vi "LeerBD.vi"(8 "error in (no error)":errorcluster) -> (0 "error out":errorcluster, 2 "BD":T1={"niv_presion_son_ref"=97.0, "Incertidumbre"="", "Tol +"="", "Tol -"="", "rangos"=[], "frecuencia_ref"=97.0}, 3 "Prueba07 out":refnum<class "Prueba07.lvclass">)   [LabVIEW 2019, in "Prueba07.lvclass"]
uses:
  Prueba07.lvclass
  BD.ctl
  Base de Datos/SQLiteConnector/SQLiteConnection.lvclass
  Base de Datos/Base de Datos.lvclass
panel:
  out "rangos out":string[][](array[string])
  in  "Tipo Equipo":enum16{"Sonometro", "Calibrador", "Dosimetro"}(ring)
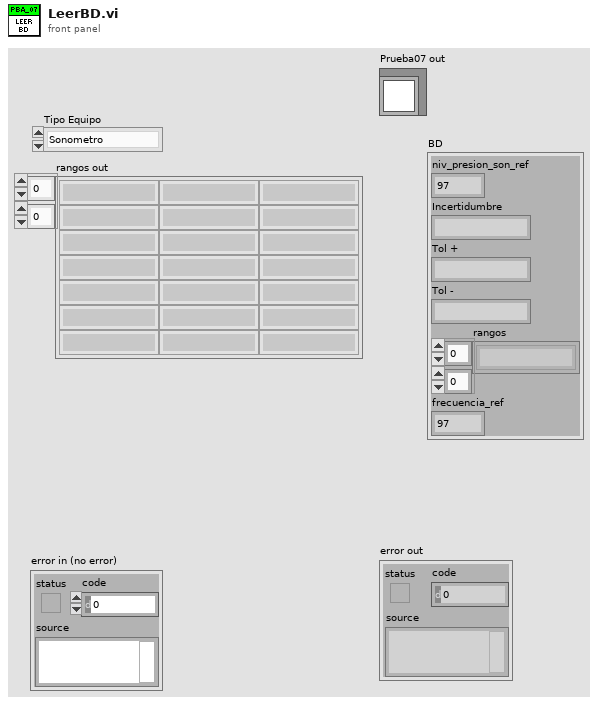
[diagram p1: front panel]
types:
  T1 = typedef "Prueba07.lvclass/BD.ctl" = cluster{"niv_presion_son_ref":dbl, "Incertidumbre":string, "Tol +":string, "Tol -":string, "rangos":string[][], "frecuencia_ref":dbl}
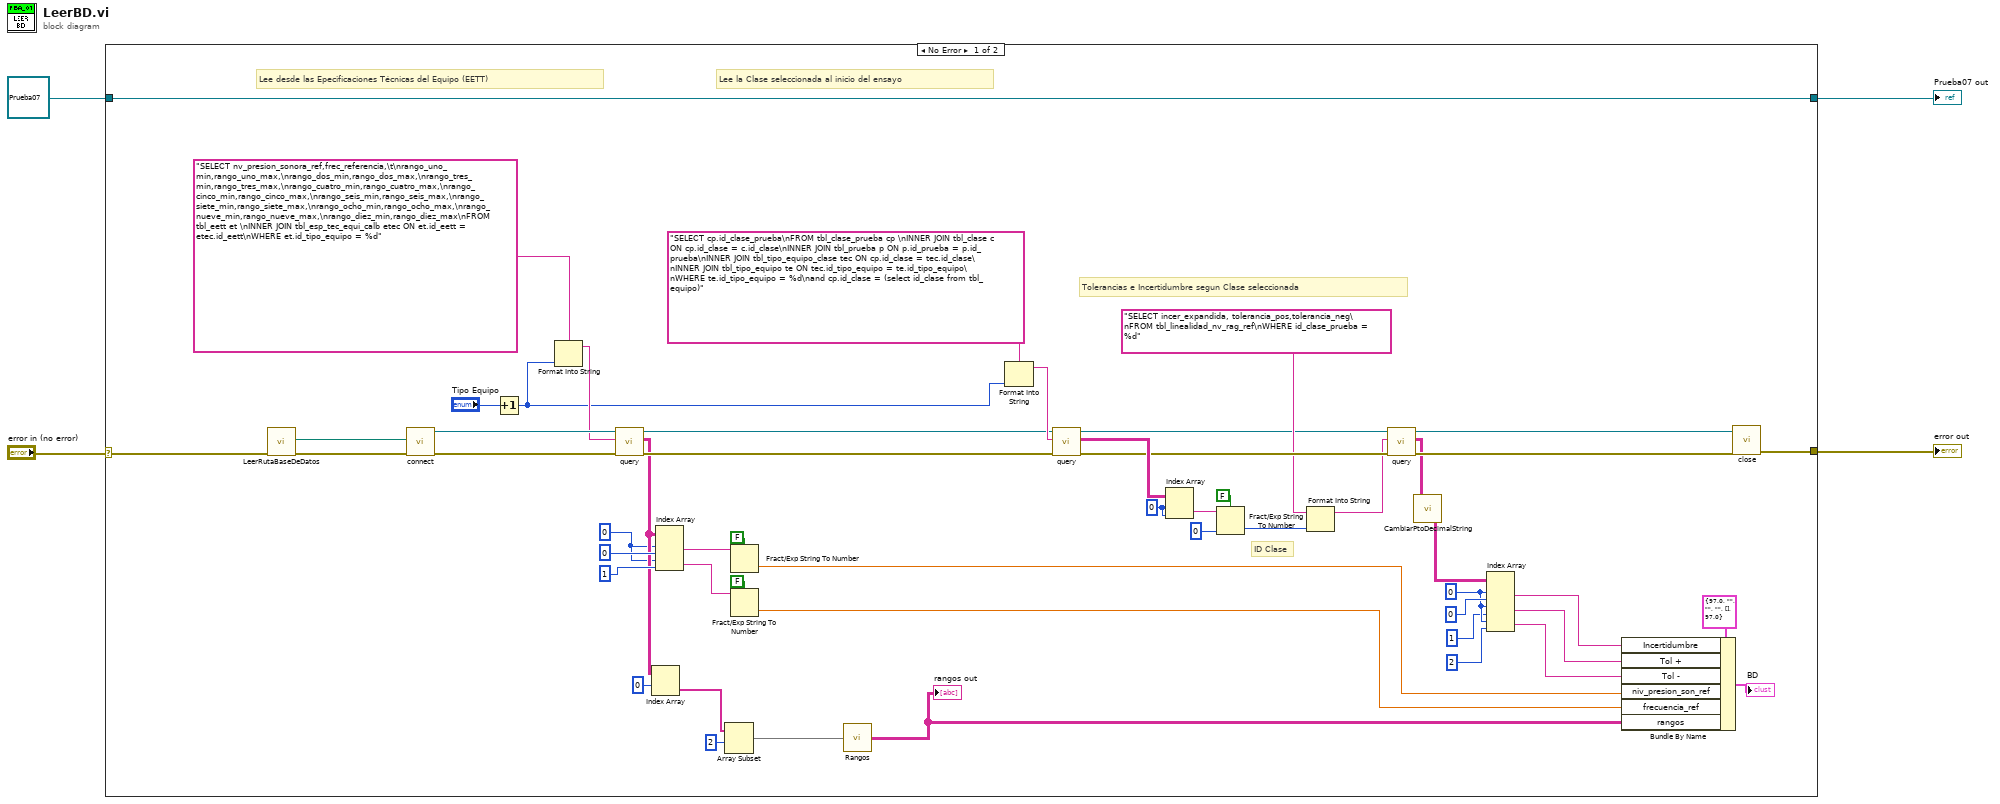
[diagram p0: block diagram]
diagram:
  n1 = case shown="No Error" "error in (no error)" {
    selector: "error in (no error)" -> [w49 w59]
    tunnel: [w35 w59] -> w3
    tunnel: [w57 w58] -> w1
    tunnel: refnum<class "Prueba07.lvclass"> refnum ("Prueba02 in") -> [w57 w58]
    frame No Error {
      w20 = 0 ("index (row)")
      w41 = 0 ("index (row)")
      w7 = 0 ("index (row)")
      # "Tolerancias e Incertidumbre segun Clase seleccionada"
      # "ID Clase"
      # "Lee la Clase seleccionada al inicio del ensayo"
      # "Lee desde las Epecificaciones Técnicas del Equipo (EETT)"
      n2 = call "LeerRutaBaseDeDatos.vi"("error in (no error)"=w49) -> ("error out"=w52:errorcluster, "Database Path"=w51:path)  [unwired: 9 in]
      n3 = call "connect.vi"("error in (no error)"=w52, "Database Path"=w51) -> ("error out"=w54:errorcluster, "object out"=w55:refnum<class "SQLiteConnection.lvclass">)  [unwired: 8 in]
      n4 = Increment(x="Tipo Equipo") -> (x+1=w30:enum16{"Sonometro", "Calibrador", "Dosimetro"})
      n5 = Format Into String(format string="SELECT nv_presion_sonora_ref,frec_referencia,\t\nrango_uno_min,rango_uno_max,\nrango_dos_min,rango_dos_max,\nrango_tres_min,rango_tres_max,\nrango_cuatro_min,rango_cuatro_max,\nrango_cinco_min,rango_cinco_max,\nrango_seis_min,rango_seis_max,\nrango_siete_min,rango_siete_max,\nrango_ocho_min,rango_ocho_max,\nrango_nueve_min,rango_nueve_max,\nrango_diez_min,rango_diez_max\nFROM tbl_eett et \nINNER JOIN tbl_esp_tec_equi_calb etec ON et.id_eett = etec.id_eett\nWHERE et.id_tipo_equipo = %d", w30) -> (resulting string=w53:string)  [unwired: 2 in, 1 out]
      n6 = call "query.vi"("error in (no error)"=w54, "SQL Statement"=w53, "object in"=w55) -> ("error out"=w42:errorcluster, "result"=w13:string[][], "object out"=w43:refnum<class "SQLiteConnection.lvclass">)  [unwired: 5 in, 1 out]
      n7 = Index Array(array=w13, index (row)=0) -> (element=w11:string[])  [unwired: 1 in]
      n8 = Index Array(array=w13, index (row) #1=w7, index (col) #1=0 ("disabled index (col)"), index (row) #2=w7, index (col) #2=1 ("disabled index (col)")) -> (element #1=w47:string, element #2=w23:string)
      n9 = Array Subset(array=w11, index=2) -> (w10:string[])  [unwired: 1 in]
      n10 = Fract/Exp String To Number(use system decimal point (T)=FALSE, string=w47) -> (number=w26:dbl)  [unwired: 2 in, 1 out]
      n11 = Fract/Exp String To Number(use system decimal point (T)=FALSE, string=w23) -> (number=w22:dbl)  [unwired: 2 in, 1 out]
      n12 = call "Rangos.vi"("rangos in"=w10) -> ("rangos out"=w6:string[][])
      "rangos out" <- w6
      n13 = Format Into String(format string="SELECT cp.id_clase_prueba\nFROM tbl_clase_prueba cp \nINNER JOIN tbl_clase c ON cp.id_clase = c.id_clase\nINNER JOIN tbl_prueba p ON p.id_prueba = p.id_prueba\nINNER JOIN tbl_tipo_equipo_clase tec ON cp.id_clase = tec.id_clase\nINNER JOIN tbl_tipo_equipo te ON tec.id_tipo_equipo = te.id_tipo_equipo\nWHERE te.id_tipo_equipo = %d\nand cp.id_clase = (select id_clase from tbl_equipo)", w30) -> (resulting string=w44:string)  [unwired: 2 in, 1 out]
      n14 = call "query.vi"("error in (no error)"=w42, "SQL Statement"=w44, "object in"=w43) -> ("error out"=w36:errorcluster, "result"=w37:string[][], "object out"=w32:refnum<class "SQLiteConnection.lvclass">)  [unwired: 5 in, 1 out]
      n15 = Index Array(array=w37, index (row)=w41, index (col)=w41) -> (element=w39:string)
      n16 = Fract/Exp String To Number(use system decimal point (T)=FALSE, string=w39, default (0 dbl)=0 ("index (row)")) -> (number=w27:i32)  [unwired: 1 in, 1 out]
      n17 = Format Into String(format string="SELECT incer_expandida, tolerancia_pos,tolerancia_neg\nFROM tbl_linealidad_nv_rag_ref\nWHERE id_clase_prueba = %d", w27) -> (resulting string=w31:string)  [unwired: 2 in, 1 out]
      n18 = call "query.vi"("error in (no error)"=w36, "SQL Statement"=w31, "object in"=w32) -> ("error out"=w33:errorcluster, "result"=w29:string[][], "object out"=w28:refnum<class "SQLiteConnection.lvclass">)  [unwired: 5 in, 1 out]
      n19 = call "CambiarPtoDecimalString.vi"("result"=w29) -> ("result out"=w5:string[][])
      n20 = Index Array(array=w5, index (row) #1=w20, index (col) #1=0 ("disabled index (col)"), index (row) #2=w20, index (col) #2=1 ("disabled index (col)"), index (row) #3=w20, index (col) #3=2 ("disabled index (col)")) -> (element #1=w17:string, element #2=w16:string, element #3=w15:string)
      n21 = Bundle By Name(cluster=T1 {"niv_presion_son_ref"=97.0, "Incertidumbre"="", "Tol +"="", "Tol -"="", "rangos"=[], "frecuencia_ref"=97.0} ("BD"), "Incertidumbre"=w17, "Tol +"=w16, "Tol -"=w15, "niv_presion_son_ref"=w26, "frecuencia_ref"=w22, "rangos"=w6) -> (→"BD":T1)
      n22 = call-dynamic "close.vi"("error in (no error)"=w33, "object in"=w28) -> ("error out"=w35:errorcluster)  [unwired: 8 in, 1 out]
    }
    frame Error {
    }
  }
  "error out" <- w3
  "Prueba07 out" <- w1
